vi "computer.vi"(8 "buf block style":u8[](array[numeric]), 10 "Layer":u8, 11 "input plate":u8[][](array[numeric])) -> (0 "Highest":i32, 3 "record":T1)   [LabVIEW 2024]
panel:
  out "All buf style":i32[](array[numeric])=[0, 1, 2, 3, 4]
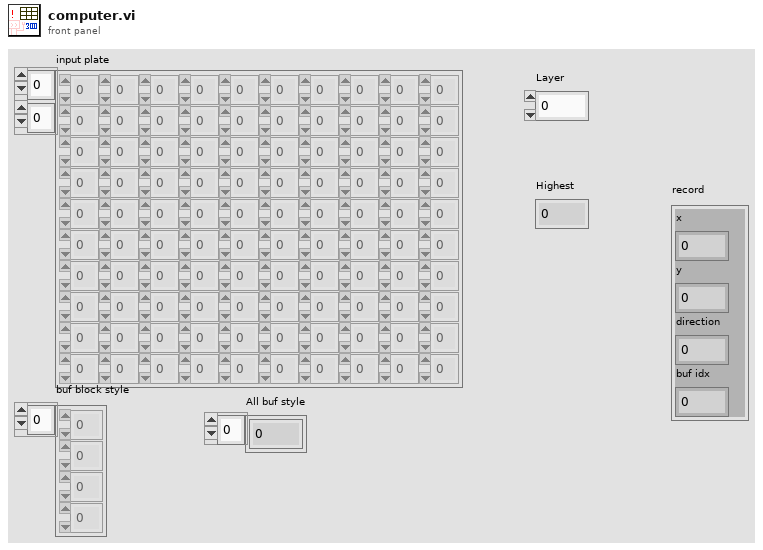
[diagram p1: front panel]
types:
  T1 = cluster{"x":u8, "y":u8, "direction":u8, "buf idx":u8}
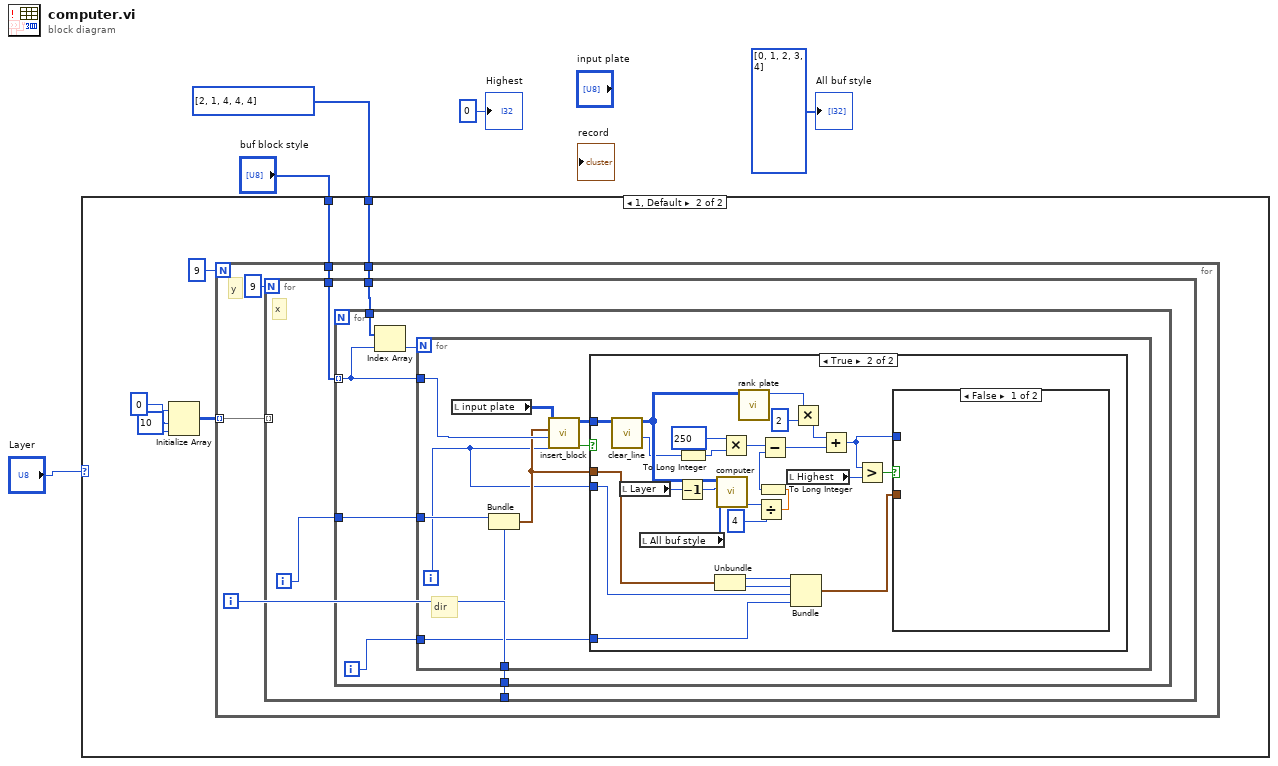
[diagram p0: block diagram]
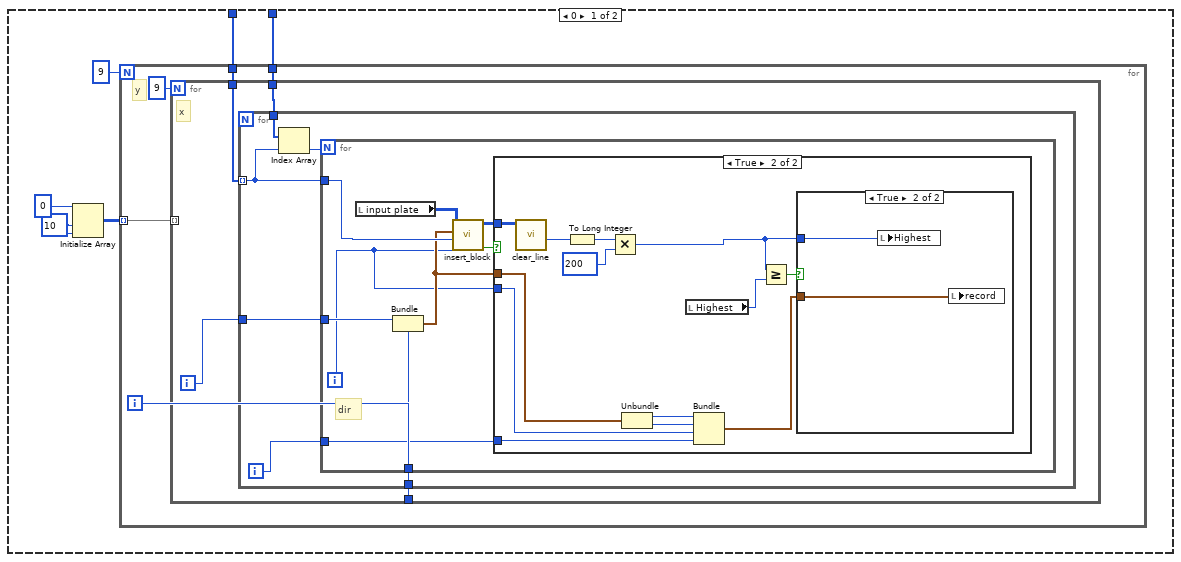
[diagram p2: hidden frame]
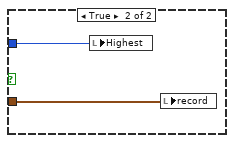
[diagram p6: hidden frame]
diagram:
  n1 = case shown="1, Default" "Layer" {
    tunnel: u16[] [2, 1, 4, 4, 4] -> [w7 w52]
    tunnel: "buf block style" -> [w6 w51]
    frame 0 {
      w11 = 10 ("dimension size")
      n2 = Initialize Array(u32 0 ("element"), w11, w11) -> (w8:u32[][])
      n3 = for {
        N: 9 -> [_]
        tunnel: w8 -> [w15] mode=indexing
        tunnel: w7 -> [w13]
        tunnel: w6 -> [w12]
        i -> [w14]
        # "y"
        n4 = for {
          N: 9 -> [_]
          tunnel: w15 -> [_] mode=indexing
          tunnel: w14 -> [w19]
          tunnel: w13 -> [w18]
          tunnel: w12 -> [w17]
          i -> [w20]
          # "x"
          n5 = for {
            tunnel: w20 -> [w26]
            tunnel: w19 -> [w25]
            tunnel: w17 -> [w23] mode=indexing
            tunnel: w18 -> [w24]
            i -> [w21]
            n6 = Index Array(array=w24, index=w23) -> (element=w22:u16)
            n7 = for {
              N: w22 -> [_]
              tunnel: w26 -> [w34]
              tunnel: w25 -> [w33]
              tunnel: w23 -> [w31]
              tunnel: w21 -> [w27]
              i -> [w28]
              # "dir"
              n8 = local read "input plate"() -> (w35:u8[][])
              n9 = Bundle(w34, w33) -> (w29:cluster{i32, i32})  [unwired: 1 in]
              n10 = call "insert_block.vi"("direction"=w28, "block_type"=w31, "position"=w29, "plate arr"=w35) -> ("valid?"=w32:bool, "return plate"=w30:u8[][])  [unwired: 6 in]
              n11 = case shown="True" w32 {
                tunnel: w28 -> [_ w40]
                tunnel: w30 -> [_ w48]
                tunnel: w29 -> [_ w41]
                tunnel: w27 -> [_ w38]
                frame False {
                }
                frame True {
                  n12 = call "clear_line.vi"("Array in"=w48) -> ("得分"=w47:u32)  [unwired: 8 in, 2 out]
                  n13 = To Long Integer(number=w47) -> (32bit integer=w37:i32)
                  n14 = Multiply(x=w37, y=200) -> (x*y=w36:i32)
                  n15 = Unbundle(w41) -> (w43:i32, w42:i32)
                  n16 = local read "Highest"() -> (w45:i32)
                  n17 = Bundle(w43, w42, w40, w38) -> (w39:cluster{i32, i32, i32, i32})  [unwired: 1 in]
                  n18 = Greater Or Equal?(x=w36, y=w45) -> (x >= y?=w44:bool)
                  n19 = case shown="True" w44 {
                    tunnel: w36 -> [_ w50]
                    tunnel: w39 -> [_ w49]
                    frame False {
                    }
                    frame True {
                      n20 = local write "Highest"(w50) -> ()
                      n21 = local write "record"(w49) -> ()
                    }
                  }
                }
              }
            }
          }
        }
      }
    }
    frame 1, Default {
      w53 = 10 ("dimension size")
      n22 = Initialize Array(u32 0 ("element"), w53, w53) -> (w56:u32[][])
      n23 = for {
        N: 9 -> [_]
        tunnel: w56 -> [w60] mode=indexing
        tunnel: w52 -> [w58]
        tunnel: w51 -> [w57]
        i -> [w59]
        # "y"
        n24 = for {
          N: 9 -> [_]
          tunnel: w60 -> [_] mode=indexing
          tunnel: w59 -> [w64]
          tunnel: w58 -> [w63]
          tunnel: w57 -> [w62]
          i -> [w65]
          # "x"
          n25 = for {
            tunnel: w65 -> [w71]
            tunnel: w64 -> [w70]
            tunnel: w62 -> [w68] mode=indexing
            tunnel: w63 -> [w69]
            i -> [w66]
            n26 = Index Array(array=w69, index=w68) -> (element=w67:u16)
            n27 = for {
              N: w67 -> [_]
              tunnel: w71 -> [w79]
              tunnel: w70 -> [w78]
              tunnel: w68 -> [w76]
              tunnel: w66 -> [w72]
              i -> [w73]
              # "dir"
              n28 = local read "input plate"() -> (w80:u8[][])
              n29 = Bundle(w79, w78) -> (w74:cluster{i32, i32})  [unwired: 1 in]
              n30 = call "insert_block.vi"("direction"=w73, "block_type"=w76, "position"=w74, "plate arr"=w80) -> ("valid?"=w77:bool, "return plate"=w75:u8[][])  [unwired: 6 in]
              n31 = case shown="True" w77 {
                tunnel: w73 -> [_ w98]
                tunnel: w75 -> [_ w106]
                tunnel: w74 -> [_ w99]
                tunnel: w72 -> [_ w96]
                frame False {
                }
                frame True {
                  n32 = call "clear_line.vi"("Array in"=w106) -> ("得分"=w88:u32, "Array out"=w91:u8[][])  [unwired: 8 in, 1 out]
                  n33 = local read "Layer"() -> (w93:u8)
                  n34 = local read "All buf style"() -> (w94:i32[])
                  n35 = Decrement(x=w93) -> (x-1=w92:u8)
                  n36 = To Long Integer(number=w88) -> (32bit integer=w87:i32)
                  n37 = Unbundle(w99) -> (w101:i32, w100:i32)
                  n38 = call "computer.vi"("buf block style"=w94, "Layer"=w92, "input plate"=w91) -> ("Highest"=w86:i32)  [unwired: 7 in, 1 out]
                  n39 = Multiply(x=250 ("y"), y=w87) -> (x*y=w90:i32)
                  n40 = call "rank plate.vi"("plate arr"=w91) -> ("total point of plate"=w105:i32)  [unwired: 10 in]
                  n41 = Divide(x=w86, y=4) -> (x/y=w84:dbl)
                  n42 = To Long Integer(number=w84) -> (32bit integer=w83:i32)
                  n43 = Subtract(x=w90, y=w83) -> (x-y=w95:i32)
                  n44 = local read "Highest"() -> (w104:i32)
                  n45 = Bundle(w101, w100, w98, w96) -> (w97:cluster{i32, i32, i32, i32})  [unwired: 1 in]
                  n46 = Multiply(x=w105, y=2) -> (x*y=w82:i32)
                  n47 = Add(x=w82, y=w95) -> (x+y=w102:i32)
                  n48 = Greater?(x=w102, y=w104) -> (0:w103:bool)
                  n49 = case shown="False" w103 {
                    tunnel: w102 -> [_ w108]
                    tunnel: w97 -> [_ w107]
                    frame False {
                    }
                    frame True {
                      n50 = local write "Highest"(w108) -> ()
                      n51 = local write "record"(w107) -> ()
                    }
                  }
                }
              }
            }
          }
        }
      }
    }
  }
  "Highest" <- 0 ("Highest")
  "All buf style" <- i32[] [0, 1, 2, 3, 4]
